vi "XYGraphs.vi"() -> ()   [LabVIEW 2024]
panel:
  out "XY Graph 2":cluster{i32[], dbl[]}(graph)
  out "XY Graph":cluster{i32[], dbl[]}(graph)
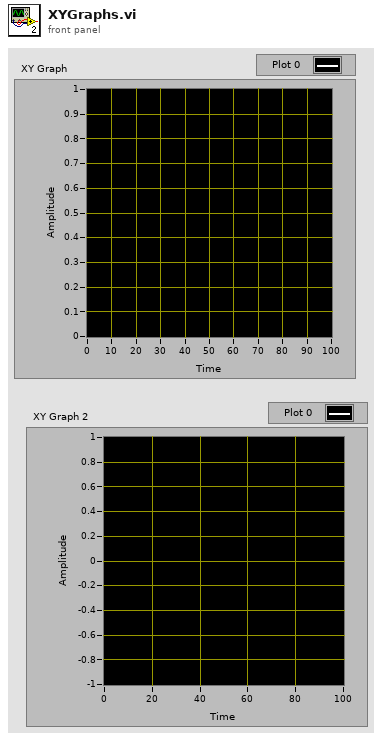
[diagram p1: front panel]
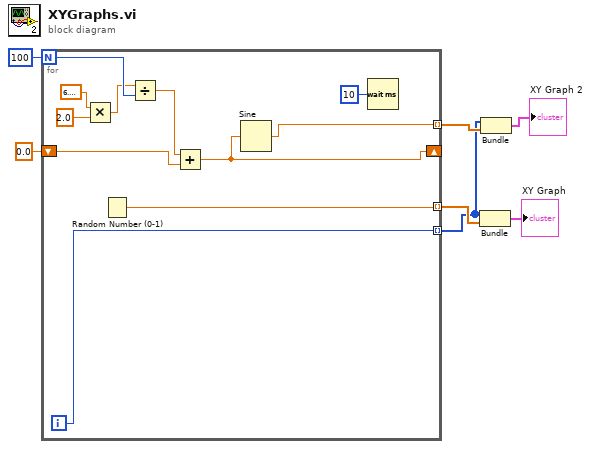
[diagram p0: block diagram]
diagram:
  n1 = for {
    N: 100 -> [w15]
    tunnel: [w18] -> w5 mode=indexing
    tunnel: [w16] -> w3 mode=indexing
    shift-right: [w12] -> _
    shift-left: 0.0 -> [w13]
    tunnel: [w11] -> w4 mode=indexing
    i -> [w16]
    n2 = Multiply(x=6.283185307179586, y=2.0) -> (x*y=w9:dbl)
    n3 = Random Number (0-1)() -> (number: 0 to 1=w18:dbl)
    n4 = Divide(x=w9, y=w15) -> (x/y=w14:dbl)
    n5 = Add(x=w14, y=w13) -> (x+y=w12:dbl)
    n6 = Sine(x=w12) -> (sin(x)=w11:dbl)
    n7 = Wait (ms)(milliseconds to wait=u32 10) -> ()  [unwired: 1 out]
  }
  n8 = Bundle(w3, w5) -> (→"XY Graph":cluster{i32[], dbl[]})  [unwired: 1 in]
  n9 = Bundle(w3, w4) -> (→"XY Graph 2":cluster{i32[], dbl[]})  [unwired: 1 in]
